vi "Show_Window_ARGB.vi"(8 "error in (no error)":errorcluster, 9 "Wait for Key (ms) (Default 0: wait forever)":i32, 10 "Window Name":string, 11 "ARGB Image":refnum<data-value>) -> (0 "error out":errorcluster, 3 "ARGB Image (duplicate)":refnum<data-value>)   [LabVIEW 2020, in "g_ar_toolkit.lvlib"]
uses:
  g_ar_toolkit.lvlib
  g_ar_toolkit.32.dll
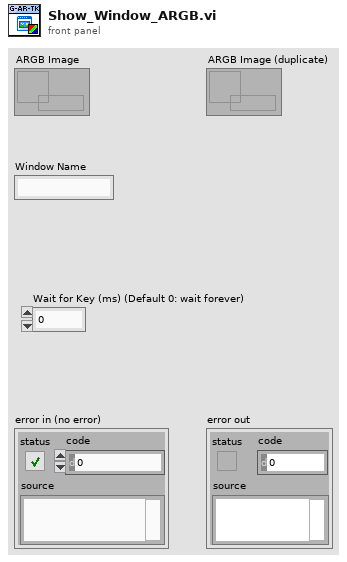
[diagram p1: front panel]
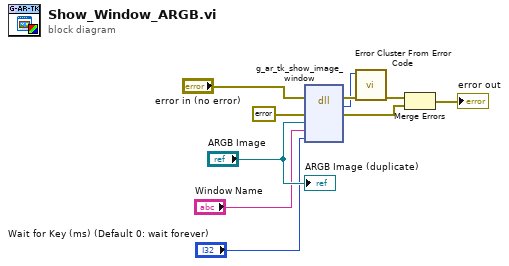
[diagram p0: block diagram]
diagram:
  n1 = dll-call lib="C:/serenial/libraries/g-augmented-reality-toolkit/LabVIEW/g_ar_toolkit/g_ar_toolkit.*.*" fn="g_ar_tk_show_image_window"(error in="error in (no error)", "error_cluster"=errorcluster {"status"=FALSE, "code"=0, "source"=""} ("error constant"), "EDVR"="ARGB Image", "window_name"="Window Name", "wait_ms"="Wait for Key (ms) (Default 0: wait forever)") -> (error out=w10:errorcluster, "MgErr"=w9:i32, "error_cluster"=w4:errorcluster)  [unwired: 5 in, 1 out]
  n2 = call <vilib>:"Error Cluster From Error Code.vi"("error in (no error)"=w10, "error code (0)"=w9) -> ("error out"=w8:errorcluster)  [unwired: 7 in]
  n3 = Merge Errors(w8, w4) -> (→"error out":errorcluster)
  "ARGB Image (duplicate)" <- "ARGB Image"
